vi "TwUpdateUserData.vi"(1 "error in (no error)":errorcluster, 2 "data":dbl[](array[numeric]), 3 "nbrElements":i32, 4 "location":string) -> (0 "error out":errorcluster)   [LabVIEW 2009]
uses:
  TofDaqDll.dll
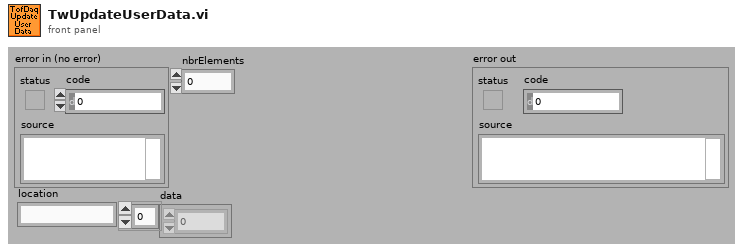
[diagram p1: front panel]
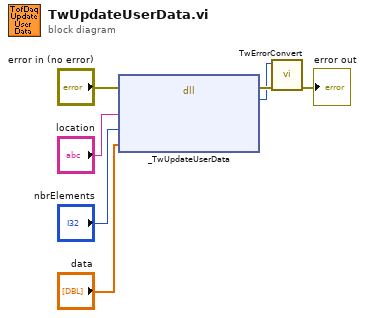
[diagram p0: block diagram]
diagram:
  n1 = dll-call lib="C:/src/TofDaq/APIandWrappers/LabView/TofDaqDll/TofDaqDll.dll" fn="_TwUpdateUserData"(error in="error in (no error)", "location"="location", "nbrElements"="nbrElements", "data"="data") -> (error out=w6:errorcluster, "TwRetVal"=w4:i32)  [unwired: 5 in, 1 out]
  n2 = call "TwErrorConvert.vi"("error in (no error)"=w6, "error code"=w4) -> ("error out"=→"error out":errorcluster)  [unwired: 9 out]
